vi "menu-ReplaceDotToSlash.vi"(11 "Array in":T1[](array[typedef])) -> (3 "Array out":T1[](array[typedef]))   [LabVIEW 2017, in "menu-operation.lvlib"]
uses:
  menu-operation.lvlib
  <resource>/Framework/Providers/API/mxLvMenuItem.ctl
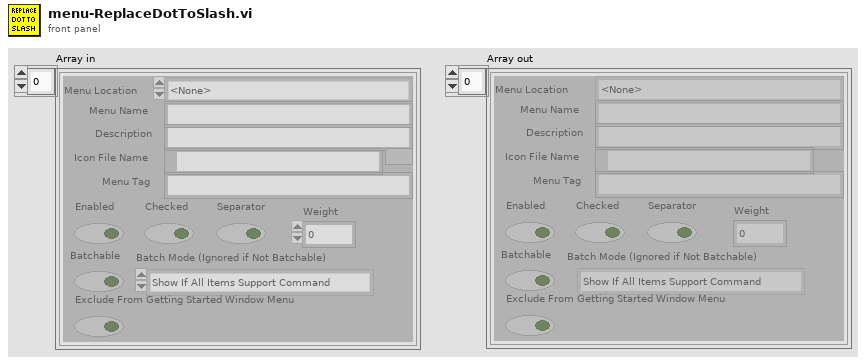
[diagram p1: front panel]
types:
  T1 = typedef "mxLvMenuItem.ctl" = cluster{"Menu Name":string, "Description":string, "Icon File Name":path, "Menu Tag":string, "Enabled":bool, "Checked":bool, "Separator":bool, "Batchable":bool, "Weight":i32, "Batch Mode (Ignored if Not Batchable)":enum32{"Show If All Items Support Command", "Show If Any Items Support Command"}, "Menu Location":enum32{"<None>", "Project", "Project / Build Specifications", "Tools", "Tools / Source Control", "Tools / Real-Time Module", "Help"}, "Exclude From Getting Started Window Menu":bool}
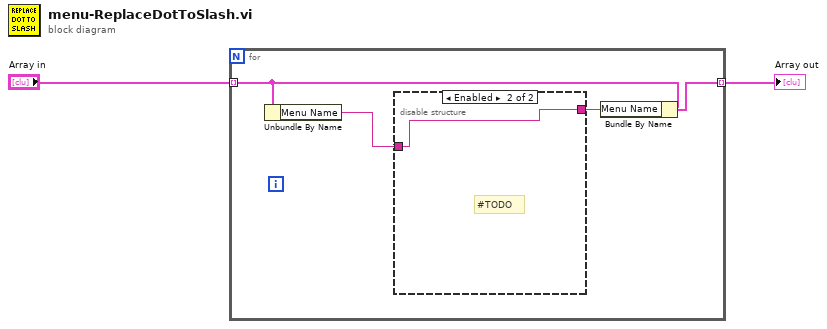
[diagram p0: block diagram]
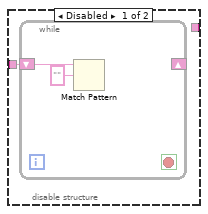
[diagram p2: hidden frame]
diagram:
  n1 = for {
    tunnel: "Array in" -> [w5] mode=indexing
    tunnel: [w6] -> w1 mode=indexing
    n2 = Unbundle By Name(w5) -> ("Menu Name"=w4:string)
    n3 = disable-structure shown="Enabled" {
      disable-tunnel: w4 -> [w7 w10]
      disable-tunnel: [_ w10] -> w3
      frame Disabled {
        n4 = while {
          shift-right: _ -> [_]
          shift-left: w7 -> [w9]
          stop <- _ stop-if-true
          n5 = Match Pattern(string=w9, regular expression="") -> ()  [unwired: 1 in, 4 out]
        }
      }
      frame Enabled {
        # "#TODO"
      }
    }
    n6 = Bundle By Name(cluster=w5, "Menu Name"=w3) -> (w6:T1)
  }
  "Array out" <- w1
